vi "iV programa 3_2.vi"() -> ()   [LabVIEW 2020]
uses:
  <vilib>/Analysis/Matrix/Numeric/Conversions/Array To Matrix - RA.vi
  <vilib>/measure/NI_MABase.lvlib
  <vilib>/Analysis/Matrix/NI_Matrix.lvlib
panel:
  out "max value sin(wt)":dbl
  out "señal senoidal y señal triangular":waveform(dbl)[](graph)
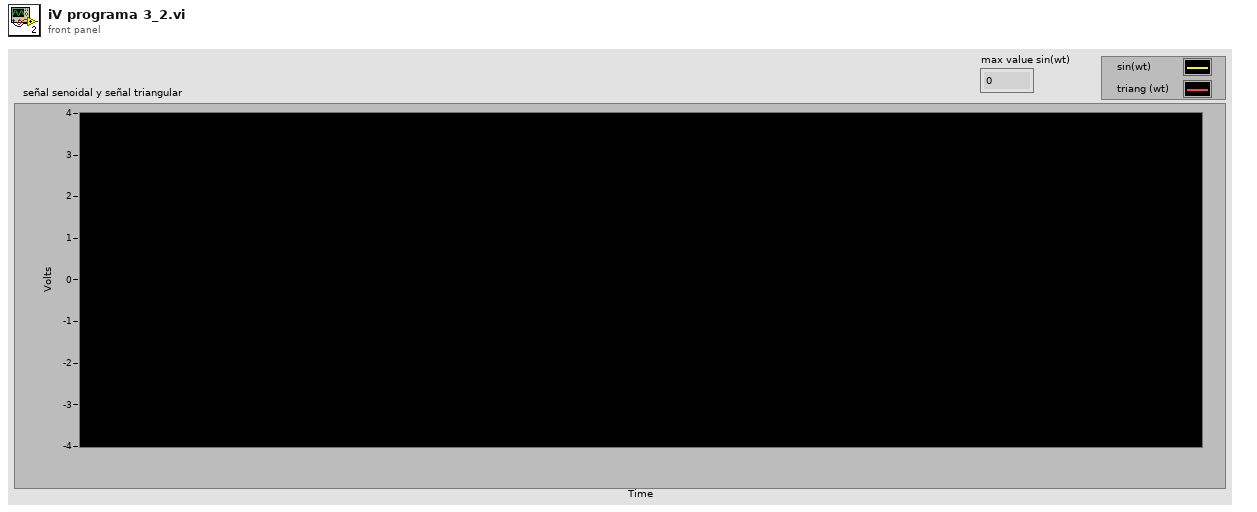
[diagram p1: front panel]
types:
  T1 = cluster{"signal out":waveform(dbl), "signal out":waveform(dbl)}
  T2 = typedef "NI_Matrix.lvlib/RealMatrix.ctl" = dbl[][]
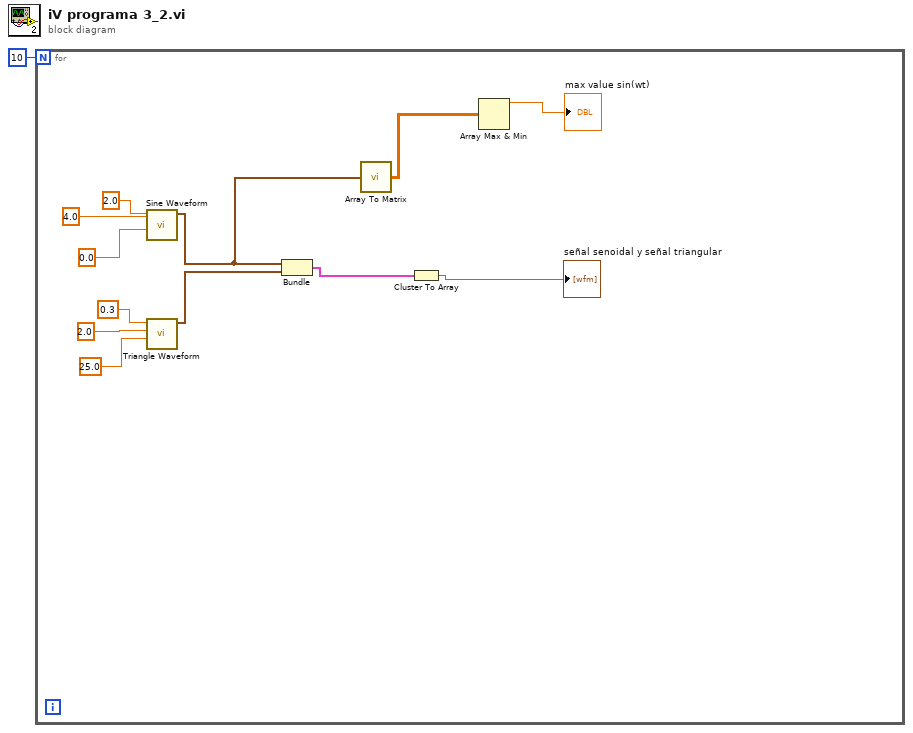
[diagram p0: block diagram]
diagram:
  n1 = for {
    N: 10 -> [_]
    n2 = call <vilib>:"Sine Waveform.vi"("phase"=0.0, "amplitude"=4.0, "frequency"=2.0) -> ("signal out"=w5:waveform(dbl))  [unwired: 7 in, 1 out]
    n3 = call <vilib>:"Triangle Waveform.vi"("phase"=25.0, "amplitude"=2.0, "frequency"=0.3) -> ("signal out"=w13:waveform(dbl))  [unwired: 7 in, 1 out]
    n4 = Bundle("signal out"=w5, "signal out"=w13) -> (w12:T1)  [unwired: 1 in]
    n5 = call-poly <vilib>:"Array To Matrix.vi"("Real 1D Array"=w5) -> ("Real Matrix (Column Vector)"=w4:T2)
    n6 = Cluster To Array(cluster=w12) -> (array=→"señal senoidal y señal triangular":waveform(dbl)[])
    n7 = Array Max & Min(array=w4) -> (max value=→"max value sin(wt)":dbl)  [unwired: 3 out]
  }
